vi "Set TreeView Column Width.vi"(8 "error in (no error)":errorcluster, 11 "TreeControl in":refnum<vi>) -> (0 "error out":errorcluster)   [LabVIEW 2018]
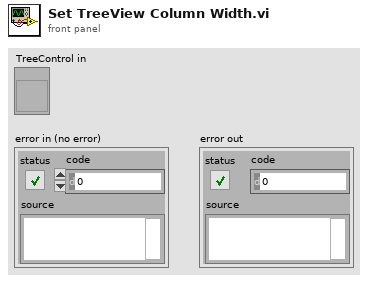
[diagram p1: front panel]
types:
  T1 = cluster{"left":i16, "top":i16, "right":i16, "bottom":i16}
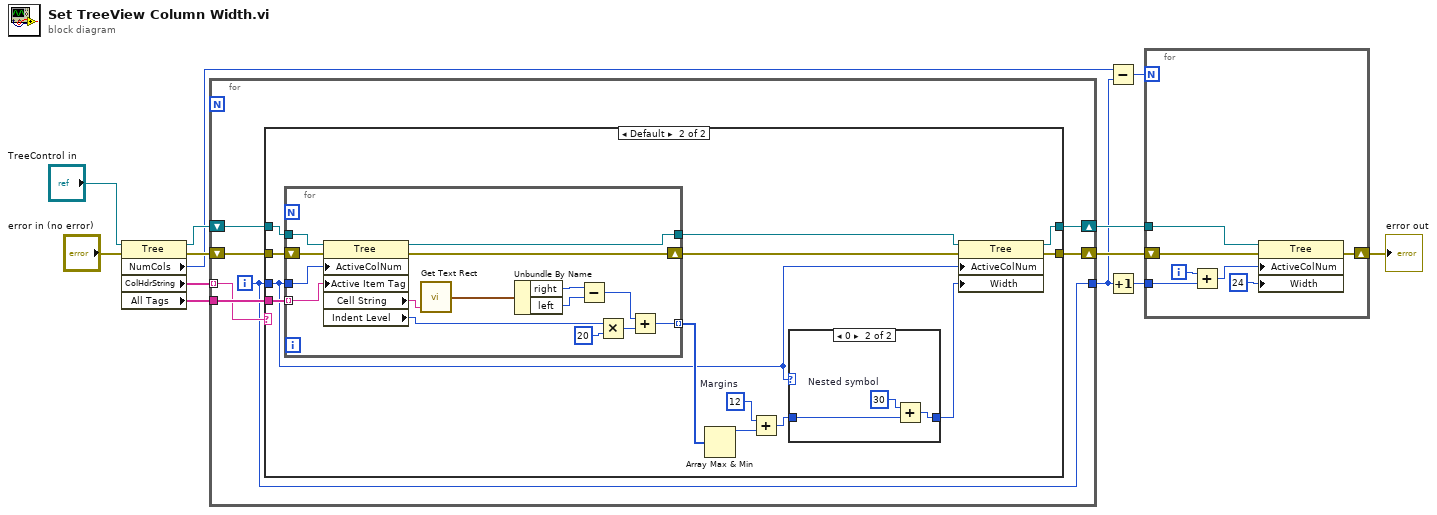
[diagram p0: block diagram]
diagram:
  n1 = property class="Tree"(reference="TreeControl in", error in="error in (no error)") -> (reference out=w11:refnum<vi>, error out=w9:errorcluster, "NumCols"=w4:u32, "ColHdrString"=w13:string[], "All Tags"=w8:string[])
  n2 = for {
    tunnel: w8 -> [w20]
    shift-right: [w17] -> w7
    shift-left: w9 -> [w19]
    tunnel: w13 -> [w16] mode=indexing
    shift-right: [w15] -> w5
    shift-left: w11 -> [w18]
    tunnel: [w14] -> w2
    i -> [w14]
    n3 = case shown="Default" w16 {
      tunnel: w20 -> [_ w35]
      tunnel: w19 -> [w22 w33]
      tunnel: w18 -> [w21 w32]
      tunnel: w14 -> [_ w28]
      tunnel: [w22 w29] -> w17
      tunnel: [w21 w23] -> w15
      frame "" {
      }
      frame Default {
        w24 = i16 12  # Margins
        n4 = for {
          tunnel: w28 -> [w54]
          tunnel: w35 -> [w53] mode=indexing
          tunnel: [w41] -> w34 mode=indexing
          tunnel: w32 -> [w46]
          tunnel: [w45] -> w31
          shift-right: [w44] -> w30
          shift-left: w33 -> [w47]
          n5 = property class="Tree"(reference=w46, error in=w47, "ActiveColNum"=w54, "Active Item Tag"=w53) -> (reference out=w45:refnum<vi>, error out=w44:errorcluster, "Cell String"=w52:string, "Indent Level"=w43:i32)
          n6 = call <vilib>:"Get Text Rect.vi"("text"=w52) -> ("rect"=w51:T1)  [unwired: 8 in]
          n7 = Unbundle By Name(w51) -> ("right"=w50:i16, "left"=w49:i16)
          n8 = Subtract(x=w50, y=w49) -> (x-y=w48:i16)
          n9 = Multiply(x=w43, y=20) -> (x*y=w40:i32)
          n10 = Add(x=w48, y=w40) -> (x+y=w41:i32)
        }
        n11 = Array Max & Min(array=w34) -> (max value=w26:i32)  [unwired: 3 out]
        n12 = Add(x=w24, y=w26) -> (x+y=w25:i32)
        n13 = case shown="0" w28 {
          tunnel: [w36 w38] -> w27
          tunnel: w25 -> [w36 w39]
          frame Default {
          }
          frame 0 {
            w37 = i16 30  # Nested symbol
            n14 = Add(x=w37, y=w39) -> (x+y=w38:i32)
          }
        }
        n15 = property class="Tree"(reference=w31, error in=w30, "ActiveColNum"=w28, "Width"=w27) -> (reference out=w23:refnum<vi>, error out=w29:errorcluster)
      }
    }
  }
  n16 = Subtract(x=w4, y=w2) -> (x-y=w3:u32)
  n17 = Increment(x=w2) -> (x+1=w1:i32)
  n18 = for {
    N: w3 -> [_]
    tunnel: w5 -> [w59]
    shift-right: [w60] -> w6
    shift-left: w7 -> [w61]
    tunnel: w1 -> [w58]
    i -> [w56]
    n19 = Add(x=w56, y=w58) -> (x+y=w57:i32)
    n20 = property class="Tree"(reference=w59, error in=w61, "ActiveColNum"=w57, "Width"=24 ("Active Cell:Cell Size:Width")) -> (error out=w60:errorcluster)  [unwired: 1 out]
  }
  "error out" <- w6
